vi "Stop Core.vi"(10 "final error code":i32, 11 "Phoenix in":refnum<class "Phoenix.lvclass">) -> (3 "Phoenix out":refnum<class "Phoenix.lvclass">)   [LabVIEW 2022 SP3, in "Phoenix.lvlib" / "Phoenix.lvclass"]
doc: "(<B>Filename</B>: Actor Framework.lvlib:Actor.lvclass:Stop Core.vi)\n\nDefines what the actor does before it stops. Use the <B>final error code</B> input to determine whether the actor shut down in response to an error.\n\nBy default, this method does nothing. A descendant class may override it to define behavior, such as shutting down any processes the actor initiated in its override of the Actor Core method."
uses:
  Phoenix.lvclass
  Phoenix.lvclass/Phoenix.ctl
  <vilib>/MGI/Monitored Actor/Monitored Actor/Monitored Actor/Monitored Actor.lvclass
  <vilib>/ActorFramework/Stop Msg/Stop Msg.lvclass
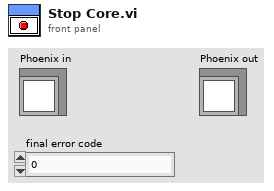
[diagram p1: front panel]
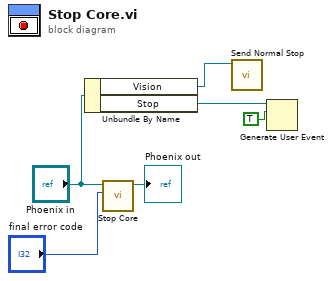
[diagram p0: block diagram]
diagram:
  n1 = Unbundle By Name("Phoenix in") -> ("Vision"=w1:refnum<class "Message Enqueuer.lvclass">, "Stop"=w3:refnum<user-event>)
  n2 = call-parent "Stop Core.vi"("final error code"="final error code", "Monitored Actor in"="Phoenix in") -> ("Monitored Actor out"=→"Phoenix out":refnum<class "Phoenix.lvclass">)  [unwired: 9 in]
  n3 = call <vilib>:"Send Normal Stop.vi"("Message Enqueuer"=w1) -> ()  [unwired: 10 in, 1 out]
  n4 = Generate User Event(user event=w3, event data cluster=TRUE ("event data")) -> ()  [unwired: 2 in, 2 out]
